vi "Test Constructor.vi"(8 "error in":errorcluster, 11 "data":T1) -> (0 "error out":errorcluster, 3 "MeasurementContext out":refnum<class "MeasurementContext.lvclass">)   [LabVIEW 2020, in "MeasurementLink Measurement Server.lvlib" / "MeasurementContext.lvclass"]
uses:
  MeasurementContext.lvclass
  Helpers/TypeDefs/PinMapContext.ctl
  MeasurementLink Measurement Server.lvlib
  <vilib>/gRPC/LabVIEW gRPC Library/Shared/grpcId.ctl
  <vilib>/gRPC/LabVIEW gRPC Library/grpc-lvsupport-release.lvlib
  IMeasurementService/IMeasurementService.lvclass
  Measurement Plugin Service/Measurement Plugin Service.lvclass
  MeasurementLink Session Management Client/RPC Messages/ni_measurementlink_sessionmanagement_v1_ChannelMapping.ctl
  MeasurementLink Session Management Client/MeasurementLink Session Management Client.lvlib
  MeasurementLink Session Management Client/RPC Messages/nidevice_grpc_Session.ctl
  MeasurementLink Session Management Client/RPC Messages/ni_measurementlink_sessionmanagement_v1_SessionInformation.ctl
  Data.ctl
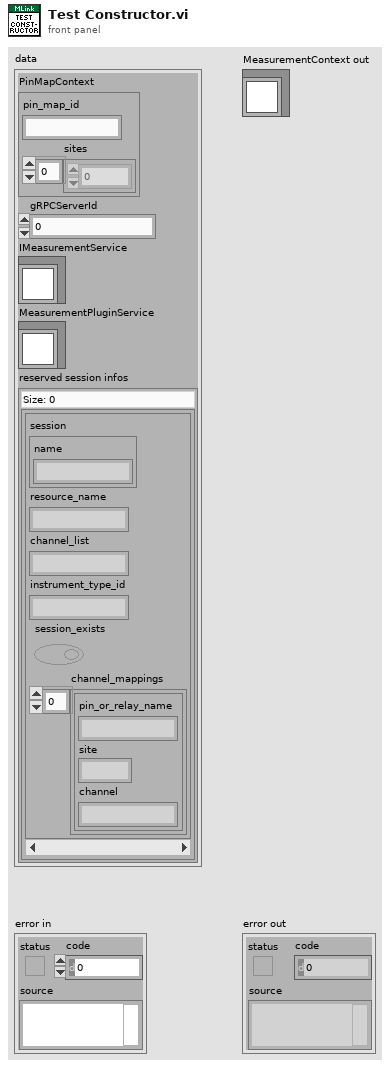
[diagram p1: front panel]
types:
  T1 = typedef "MeasurementLink Measurement Server.lvlib/MeasurementContext.lvclass/Data.ctl" = cluster{"PinMapContext":T2, "gRPCServerId":T3, "IMeasurementService":refnum<class "IMeasurementService.lvclass">, "MeasurementPluginService":refnum<class "Measurement Plugin Service.lvclass">, "reserved session infos":set{T4}}
  T2 = typedef "MeasurementLink Measurement Server.lvlib/PinMapContext.ctl" = cluster{"pin_map_id":string, "sites":i32[]}
  T3 = typedef "grpc-lvsupport-release.lvlib/grpcId.ctl" = u64
  T4 = typedef "MeasurementLink Session Management Client.lvlib/ni_measurementlink_sessionmanagement_v1_SessionInformation.ctl" = cluster{"session":T5, "resource_name":string, "channel_list":string, "instrument_type_id":string, "session_exists":bool, "channel_mappings":T6[]}
  T5 = typedef "MeasurementLink Session Management Client.lvlib/nidevice_grpc_Session.ctl" = cluster{"name":string}
  T6 = typedef "MeasurementLink Session Management Client.lvlib/ni_measurementlink_sessionmanagement_v1_ChannelMapping.ctl" = cluster{"pin_or_relay_name":string, "site":i32, "channel":string}
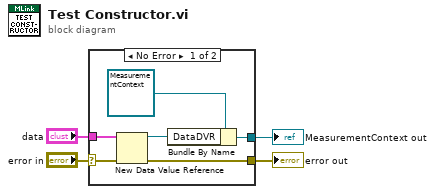
[diagram p0: block diagram]
diagram:
  n1 = case shown="No Error" "error in" {
    selector: "error in" -> [w10 w11]
    tunnel: [w5 w11] -> w3
    tunnel: [w9 _] -> w2
    tunnel: "data" -> [w7 _]
    frame No Error {
      n2 = New Data Value Reference(data value=w7, error in=w10) -> (data value reference=w6:refnum<data-value>, error out=w5:errorcluster)
      n3 = Bundle By Name(cluster=refnum<class "MeasurementContext.lvclass"> refnum ("MeasurementContext in"), "DataDVR"=w6) -> (w9:refnum<class "MeasurementContext.lvclass">)
    }
    frame Error {
    }
  }
  "error out" <- w3
  "MeasurementContext out" <- w2
